vi "1B_HiStim_AnalyzePulseTrain.vi"(0 "Waveform In":waveform(dbl)={"t0"=timestamp(3433165898.5470004 s since 1904-01-01), "dt"=1e-05, "Y"=array[4250 elements]}, 5 "Repetitions in the Input Waveform":i32, 7 "Pulse Characteristics":T1={"Pulses per Cycle"=2, "Load Resistance (Ohms)"=750.0, "Krec Value"=2, "Recovery Mode (T=Active)"=TRUE, "Target Stim Currents (Amps)"=[]} {"Target Stim Currents (Amps)" format="%#_6p"}) -> (2 "Avg. CBC Width":dbl format="%0.6f", 3 "Avg. CBC Amplitude":dbl format="%0.2f", 4 "Stim PW":dbl[](array[numeric]), 6 "Stim Amplitude":dbl[](array[numeric]), 8 "Interphase Delay":dbl[](array[numeric]), 10 "Recovery PW":dbl[](array[numeric]), 12 "Waveform Parameters":T2 {"Frequency" format="%#_6p"; "Avg CBC Width" format="%#_6p"; "Avg. CBC Holdoff" format="%#_6p"; "Stim Pulse Width" format="%^#_6g"; "Interphase Delay" format="%#_6p"; "Recovery PW" format="%#_6p"; "Recovery Holdoff" format="%#_6p"; "Stim Amplitude" format="%^#_6g"; "Recovery Amplitude" format="%#_6p"}, 13 "Frequency":dbl, 14 "Recovery Holdoff":dbl[](array[numeric]), 15 "Recovery Amplitude":dbl[](array[numeric]))   [LabVIEW 2010]
uses:
  <vilib>/measure/mamon.llb/Trigger Detection for 1 Channel.vi
  <vilib>/measure/NI_MAPro.lvlib
  <vilib>/Analysis/NI_AALBase.lvlib
panel:
  in  "View":enum32{"View All", "Graph Only"}(tab)
  out "Waveform in ( graph )":waveform(dbl)(graph)
  out "Normalized Waveform":waveform(dbl)(graph)
  out "Offset":dbl
  out "Eq. Freq ( Hz )":dbl format="%#_6p"
  out "Current in amps":waveform(dbl)(graph)
  out "Time2 - Time1 ( sec )":dbl format="%#_6p"
  out "index":i32
  # "Remove idle voltage offset\n( if applicable )"
  # "The input waveform should be a capture of the STIM chip output\n(before the cap) when the output is held at 1/2 HVDD by the\nLoad Resistance.  This ensures that passive recovery and CBC\npulses are captured, because they look like pulses pulled to GND."
  # "The elements in these arrays correspond to the pulses per cycle.\nThey are the averages over all the repetitions in the waveform."
  # "Enter Target Current\nfor each in array below"
  # "1. Update Cursor Positions\n2. Turn off X Autoscaling\n3. Run this VI again"
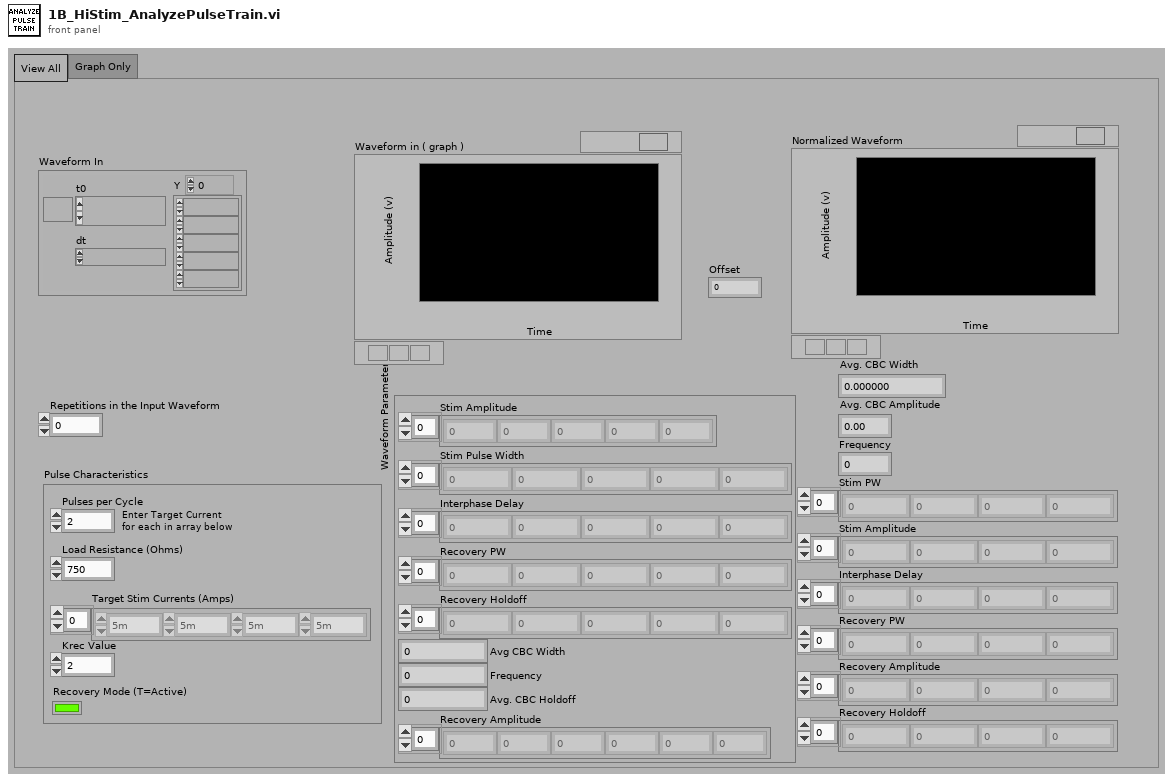
[diagram p1: front panel]
types:
  T1 = cluster{"Pulses per Cycle":i32, "Load Resistance (Ohms)":dbl, "Krec Value":i32, "Recovery Mode (T=Active)":bool, "Target Stim Currents (Amps)":dbl[]}
  T2 = cluster{"Stim Amplitude":dbl[], "Stim Pulse Width":dbl[], "Interphase Delay":dbl[], "Recovery PW":dbl[], "Recovery Holdoff":dbl[], "Avg CBC Width":dbl, "Frequency":dbl, "Avg. CBC Holdoff":dbl, "Recovery Amplitude":dbl[]}
  T3 = cluster{"trigger slope":u16, "Trigger Level":dbl}[]
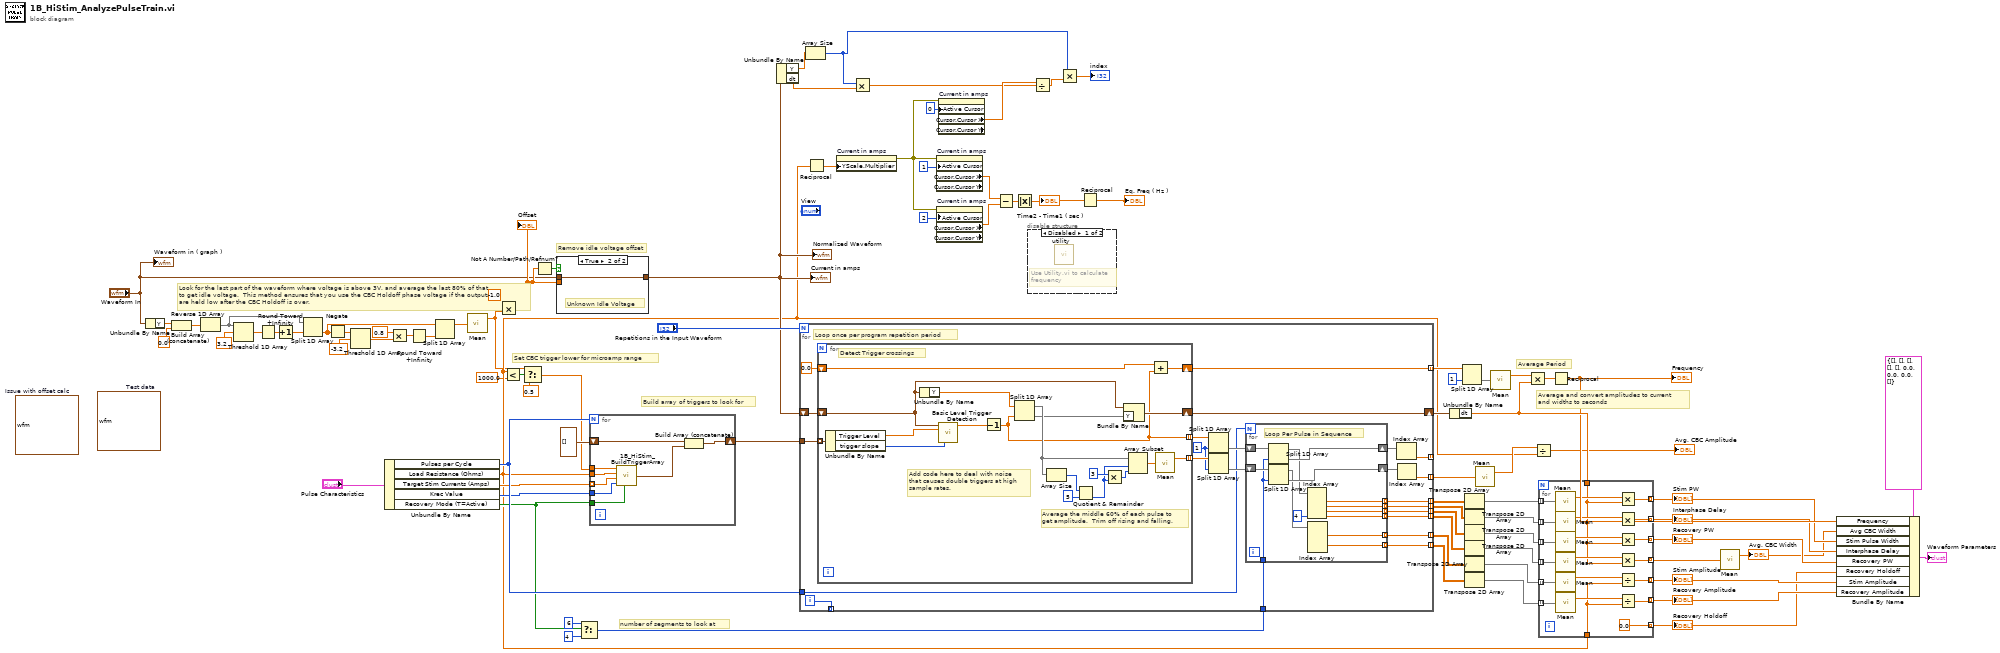
[diagram p0: block diagram]
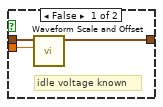
[diagram p3: hidden frame]
diagram:
  (unwired) waveform(dbl) {"t0"=timestamp(3458836317.3280005 s since 1904-01-01), "dt"=1.428e-05, "Y"=array[4000 elements]}  # Issue with offset calc
  (unwired) waveform(dbl) {"t0"=timestamp(3418839276.250478 s since 1904-01-01), "dt"=1e-06, "Y"=[5.0, 5.0, 9.0, 9.0, 9.0, 9.0, 9.0, 9.0, 9.0, 9.0, 5.0, 5.0, 5.0, 3.0, 3.0, 3.0, 3.0, 3.0, 3.0, 3.0, 3.0, 3.0, 3.0, 3.0, 3.0, 3.0, 3.0, 3.0, 3.0, 5.0, 5.0, 5.0, 5.0, 8.0, 8.0, 8.0, 8.0, 8.0, 8.0, 8.0, 8.0, 5.0, 5.0, 5.0, 3.0, 3.0, 3.0, 3.0, 3.0, 3.0, 3.0, 3.0, 3.0, 3.0, 3.0, 3.0, 3.0, 3.0, 3.0, 3.0, 5.0, 5.0, 5.0, 5.0, 0.0, 0.0, 0.0, 0.0, 0.0, 5.0, 5.0, 5.0, 5.0, 5.0, 5.0, 5.0, 5.0, 5.0, 5.0, 5.0, 5.0, 5.0, 5.0, 5.0, 5.0, 5.0, 5.0, 5.0, 5.0, 5.0, 5.0, 5.0, 5.0, 5.0, 5.0, 5.0, 5.0, 5.0, 5.0, 5.0, 5.0, 5.0, 9.0, 9.0, 9.0, 9.0, 9.0, 9.0, 9.0, 9.0, 5.0, 5.0, 5.0, 3.0, 3.0, 3.0, 3.0, 3.0, 3.0, 3.0, 3.0, 3.0, 3.0, 3.0, 3.0, 3.0, 3.0, 3.0, 3.0, 5.0, 5.0, 5.0, 5.0, 8.0, 8.0, 8.0, 8.0, 8.0, 8.0, 8.0, 8.0, 5.0, 5.0, 5.0, 3.0, 3.0, 3.0, 3.0, 3.0, 3.0, 3.0, 3.0, 3.0, 3.0, 3.0, 3.0, 3.0, 3.0, 3.0, 3.0, 5.0, 5.0, 5.0, 5.0, 0.0, 0.0, 0.0, 0.0, 0.0, 5.0, 5.0, 5.0, 5.0, 5.0, 5.0, 5.0, 5.0, 5.0, 5.0, 5.0, 5.0, 5.0, 5.0, 5.0, 5.0, 5.0, 5.0, 5.0, 5.0, 5.0, 5.0, 5.0, 5.0, 5.0, 5.0, 5.0, 5.0, 5.0, 5.0, 5.0, 5.0, 5.0, 9.0, 9.0, 9.0, 9.0, 9.0, 9.0, 9.0, 9.0, 5.0, 5.0, 5.0, 3.0, 3.0, 3.0, 3.0, 3.0, 3.0, 3.0, 3.0, 3.0, 3.0, 3.0, 3.0, 3.0, 3.0, 3.0, 3.0, 5.0, 5.0, 5.0, 5.0, 8.0, 8.0, 8.0, 8.0, 8.0, 8.0, 8.0, 8.0, 5.0, 5.0, 5.0, 3.0, 3.0, 3.0, 3.0, 3.0, 3.0, 3.0, 3.0, 3.0, 3.0, 3.0, 3.0, 3.0, 3.0, 3.0, 3.0, 5.0, 5.0, 5.0, 5.0, 0.0, 0.0, 0.0, 0.0, 0.0, 5.0, 5.0, 5.0, 5.0, 5.0, 5.0, 5.0, 5.0, 5.0, 5.0, 5.0, 5.0, 5.0, 5.0, 5.0, 5.0, 5.0, 5.0, 5.0, 5.0, 5.0, 5.0, 5.0, 5.0, 5.0, 5.0, 5.0, 5.0, 5.0, 5.0, 5.0, 5.0, 5.0, 9.0, 9.0, 9.0, 9.0, 9.0, 9.0, 9.0, 9.0, 5.0, 5.0, 5.0, 3.0, 3.0, 3.0, 3.0, 3.0, 3.0, 3.0, 3.0, 3.0, 3.0, 3.0, 3.0, 3.0, 3.0, 3.0, 3.0, 5.0, 5.0, 5.0, 5.0, 8.0, 8.0, 8.0, 8.0, 8.0, 8.0, 8.0, 8.0, 5.0, 5.0, 5.0, 3.0, 3.0, 3.0, 3.0, 3.0, 3.0, 3.0, 3.0, 3.0, 3.0, 3.0, 3.0, 3.0, 3.0, 3.0, 3.0, 5.0, 5.0, 5.0, 5.0, 0.0, 0.0, 0.0, 0.0, 0.0, 5.0, 5.0, 5.0, 5.0, 5.0, 5.0, 5.0, 5.0, 5.0, 5.0, 5.0, 5.0, 5.0, 5.0, 5.0, 5.0, 5.0, 5.0, 5.0, 5.0, 5.0, 5.0, 5.0, 5.0, 5.0, 5.0, 5.0, 5.0, 5.0, 5.0, 5.0, 5.0, 5.0, 9.0, 9.0, 9.0, 9.0, 9.0, 9.0, 9.0, 9.0, 5.0, 5.0, 5.0, 3.0, 3.0, 3.0, 3.0, 3.0, 3.0, 3.0, 3.0, 3.0, 3.0, 3.0, 3.0, 3.0, 3.0, 3.0, 3.0, 5.0, 5.0, 5.0, 5.0, 8.0, 8.0, 8.0, 8.0, 8.0, 8.0, 8.0, 8.0, 5.0, 5.0, 5.0, 3.0, 3.0, 3.0, 3.0, 3.0, 3.0, 3.0, 3.0, 3.0, 3.0, 3.0, 3.0, 3.0, 3.0, 3.0, 3.0, 5.0, 5.0, 5.0, 5.0, 0.0, 0.0, 0.0, 0.0, 0.0, 5.0, 5.0, 5.0, 5.0, 5.0, 5.0, 5.0, 5.0, 5.0, 5.0, 5.0, 5.0, 5.0, 5.0, 5.0, 5.0, 5.0, 5.0, 5.0, 5.0, 5.0, 5.0, 5.0, 5.0, 5.0, 5.0, 5.0, 5.0, 5.0, 5.0, 5.0, 5.0, 5.0, 5.0]}  # Test data
  # "Set CBC trigger lower for microamp range"
  # "number of segments to look at"
  # "Look for the last part of the waveform where voltage is above 3V, and average the last 80% of that\nto get idle voltage.  This method ensures that you use the CBC Holdoff phase voltage if the outputs\nare held low after the CBC Holdoff is over."
  # "Average Period"
  # "Average and convert amplitudes to current\nand widths to seconds"
  # "Build array of triggers to look for"
  # "Remove idle voltage offset"
  n1 = Unbundle By Name("Waveform In") -> ("Y"=w9:dbl[])
  n2 = Build Array (concatenate)(w9, 0.0 ("y")) -> (w8:dbl[])
  n3 = Reverse 1D Array(array=w8) -> (reversed array=w7:dbl[])
  n4 = Threshold 1D Array(2:3.2 ("y"), 3:w7) -> (0:w52:dbl)  [unwired: 1 in]
  n5 = Round Toward +Infinity(x=w52) -> (ceil(x): smallest int >= x=w51:dbl)
  n6 = Increment(x=w51) -> (x+1=w44:dbl)
  n7 = Split 1D Array(array=w7, index=w44) -> (second subarray=w32:dbl[])  [unwired: 1 out]
  n8 = Negate(x=w32) -> (-x=w49:dbl[])
  n9 = Threshold 1D Array(2:-3.2 ("y"), 3:w49) -> (0:w48:dbl)  [unwired: 1 in]
  n10 = Unbundle By Name("Pulse Characteristics") -> ("Pulses per Cycle"=w73:i32, "Load Resistance (Ohms)"=w6:dbl, "Target Stim Currents (Amps)"=w18:dbl[], "Krec Value"=w72:i32, "Recovery Mode (T=Active)"=w39:bool)
  n11 = Multiply(x=0.8, y=w48) -> (x*y=w46:dbl)
  n12 = Round Toward +Infinity(x=w46) -> (ceil(x): smallest int >= x=w45:dbl)
  n13 = Split 1D Array(array=w32, index=w45) -> (first subarray=w31:dbl[])  [unwired: 1 out]
  n14 = call <vilib>:"Mean.vi"("X"=w31) -> ("mean"=w3:dbl)  [unwired: 1 out]
  n15 = Multiply(x=-1.0, y=w3) -> (x*y=w34:dbl)
  "Offset" <- w34
  n16 = Less?(x=w6, y=1000.0) -> (x < y?=w4:bool)
  n17 = Select(t=w3, s=w4, f=0.5) -> (s? t:f=w2:dbl)
  n18 = Not A Number/Path/Refnum?(number/path/refnum=w34) -> (NaN/Path/Refnum?=w33:bool)
  n19 = case shown="True" w33 {
    tunnel: [w91 w92] -> w17
    tunnel: "Waveform In" -> [w90 w92]
    tunnel: w34 -> [w89 _]
    frame False {
      # "idle voltage known"
      n20 = call <vilib>:"Waveform Scale and Offset.vi"("offset"=w89, "waveform in"=w90) -> ("waveform out"=w91:waveform(dbl))  [unwired: 8 in, 1 out]
    }
    frame True {
      # "Unknown Idle Voltage"
    }
  }
  "Normalized Waveform" <- w17
  "Current in amps" <- w17
  n21 = Select(t=6, s=w39, f=4 ("index")) -> (s? t:f=w37:i32)
  n22 = for {
    N: w73 -> [_]
    shift-right: [w100] -> w43
    shift-left: T3 [] -> [w99]
    tunnel: w2 -> [w98]
    tunnel: w39 -> [w97]
    tunnel: w6 -> [w96]
    tunnel: w18 -> [w95] mode=indexing
    tunnel: w72 -> [w94]
    n23 = call "1B_HiStim_BuildTriggerArray.vi"("CBC Trigger Level"=w98, "Load Resistance (Ohms)"=w96, "Target Stim Current (Amps)"=w95, "Krec Value"=w94, "Recovery Mode (T=Active)"=w97) -> ("Pulse Triggers"=w93:T3)
    n24 = Build Array (concatenate)(w99, w93) -> (w100:T3)
  }
  n25 = Unbundle By Name(w17) -> ("Y"=w13:dbl[], "dt"=w12:dbl)
  n26 = for {
    N: "Repetitions in the Input Waveform" -> [_]
    tunnel: w43 -> [w123]
    shift-right: [w119] -> w70
    shift-left: w17 -> [w122]
    tunnel: w73 -> [w116]
    tunnel: [w113] -> _ mode=indexing
    tunnel: [w112] -> w86 mode=indexing
    tunnel: [w111] -> w85 mode=indexing
    tunnel: [w110] -> w84 mode=indexing
    tunnel: [w109] -> w83 mode=indexing
    tunnel: [w108] -> w82 mode=indexing
    tunnel: [w107] -> w81 mode=indexing
    tunnel: [w106] -> w80 mode=indexing
    tunnel: [w103] -> w68 mode=indexing
    tunnel: w37 -> [w102]
    tunnel: [w101] -> _ mode=indexing
    i -> [w101]
    w120 = 1 ("index")
    # "Loop once per program repetition period"
    n27 = for {
      tunnel: w123 -> [w156] mode=indexing
      shift-right: [w143] -> w119
      shift-left: w122 -> [w139]
      tunnel: [w148] -> w121 mode=indexing
      tunnel: [w141] -> w104 mode=indexing
      shift-right: [w147] -> w103
      shift-left: 0.0 -> [w146]
      # "Add code here to deal with noise \nthat causes double triggers at high\nsample rates."
      # "Detect Trigger crossings"
      # "Average the middle 60% of each pulse to\nget amplitude.  Trim off rising and falling."
      n28 = Unbundle By Name(w156) -> ("Trigger Level"=w145:dbl, "trigger slope"=w144:u16)
      n29 = Unbundle By Name(w139) -> ("Y"=w140:dbl[])
      n30 = call-poly <vilib>:"Basic Level Trigger Detection.vi"("signal in"=w139, "level"=w145, "trigger slope"=w144) -> ("trigger location"=w138:dbl)  [unwired: 10 in, 2 out]
      n31 = Decrement(x=w138) -> (x-1=w141:dbl)
      n32 = Split 1D Array(array=w140, index=w141) -> (first subarray=w150:dbl[], second subarray=w142:dbl[])
      n33 = Array Size(array=w150) -> (size(s)=w155:i32)
      n34 = Quotient & Remainder(x=w155, y=5) -> (floor(x/y)=w152:i32)  [unwired: 1 out]
      n35 = Multiply(x=3, y=w152) -> (x*y=w151:i32)
      n36 = Bundle By Name(cluster=w139, "Y"=w142) -> (w143:waveform(dbl))
      n37 = Array Subset(array=w150, index=w152, length=w151) -> (w149:dbl[])
      n38 = Add(x=w146, y=w141) -> (x+y=w147:dbl)
      n39 = call <vilib>:"Mean.vi"("X"=w149) -> ("mean"=w148:dbl)  [unwired: 1 out]
    }
    n40 = Split 1D Array(array=w104, index=w120) -> (second subarray=w118:dbl[])  [unwired: 1 out]
    n41 = Split 1D Array(array=w121, index=w120) -> (second subarray=w117:dbl[])  [unwired: 1 out]
    n42 = for {
      N: w116 -> [_]
      shift-right: [w135] -> w115
      shift-left: w118 -> [w137]
      shift-right: [w134] -> w114
      shift-left: w117 -> [w136]
      tunnel: [w131] -> w111 mode=indexing
      tunnel: [w130] -> w110 mode=indexing
      tunnel: [w129] -> w109 mode=indexing
      tunnel: [w128] -> w108 mode=indexing
      tunnel: [w127] -> w107 mode=indexing
      tunnel: [w126] -> w106 mode=indexing
      tunnel: w102 -> [w125]
      # "Loop Per Pulse in Sequence"
      n43 = Split 1D Array(array=w137, index=w125) -> (first subarray=w133:dbl[], second subarray=w135:dbl[])
      n44 = Split 1D Array(array=w136, index=w125) -> (first subarray=w132:dbl[], second subarray=w134:dbl[])
      n45 = Index Array(array=w133, index #4=4 ("index")) -> (element #1=w131:dbl, element #2=w130:dbl, element #3=w129:dbl, element #4=w128:dbl)  [unwired: 3 in]
      n46 = Index Array(array=w132) -> (element #1=w127:dbl, element #3=w126:dbl)  [unwired: 4 in, 2 out]
    }
    n47 = Index Array(array=w115) -> (element=w113:dbl)  [unwired: 1 in]
    n48 = Index Array(array=w114) -> (element=w112:dbl)  [unwired: 1 in]
  }
  n49 = Array Size(array=w13) -> (size(s)=w11:i32)
  n50 = Reciprocal(x=w6) -> (1/x=w35:dbl)
  n51 = property on="Current in amps" class="WFGraph (strict)"("YScale.Multiplier"=w35) -> (error out=w20:errorcluster)  [unwired: 2 in, 1 out]
  n52 = Multiply(x=w11, y=w12) -> (x*y=w10:dbl)
  n53 = property on="Current in amps" class="WFGraph (strict)" props=["Active Cursor", "Cursor", "Cursor X", "Cursor", "Cursor Y"](error in=w20, "Active Cursor"=u32 1) -> ("Cursor.Cursor X"=w24:dbl)  [unwired: 1 in, 3 out]
  n54 = property on="Current in amps" class="WFGraph (strict)" props=["Active Cursor", "Cursor", "Cursor X", "Cursor", "Cursor Y"](error in=w20, "Active Cursor"=u32 2) -> ("Cursor.Cursor X"=w23:dbl)  [unwired: 1 in, 3 out]
  n55 = property on="Current in amps" class="WFGraph (strict)" props=["Active Cursor", "Cursor", "Cursor X", "Cursor", "Cursor Y"](error in=w20, "Active Cursor"=u32 0) -> ("Cursor.Cursor X"=w16:dbl)  [unwired: 1 in, 3 out]
  n56 = Subtract(x=w24, y=w23) -> (x-y=w25:dbl)
  n57 = Absolute Value(x=w25) -> (abs(x)=w22:dbl)
  "Time2 - Time1 ( sec )" <- w22
  n58 = disable-structure shown="Disabled" {
    frame Disabled {
      # "Use Utility.vi to calculate\nfrequency"
      n59 = call "utility.vi"() -> ()  [unwired: 12 in]
    }
    frame Enabled {
    }
  }
  n60 = Divide(x=w16, y=w10) -> (x/y=w15:dbl)
  n61 = Multiply(x=w11, y=w15) -> (x*y=→"index":dbl)
  n62 = Reciprocal(x=w22) -> (1/x=→"Eq. Freq ( Hz )":dbl)
  n63 = Unbundle By Name(w70) -> ("dt"=w65:dbl)
  n64 = Split 1D Array(array=w68, index=1) -> (second subarray=w67:dbl[])  [unwired: 1 out]
  n65 = Transpose 2D Array(2D array=w85) -> (transposed array=w79:dbl[][])
  n66 = Transpose 2D Array(2D array=w84) -> (transposed array=w78:dbl[][])
  n67 = Transpose 2D Array(2D array=w83) -> (transposed array=w77:dbl[][])
  n68 = Transpose 2D Array(2D array=w82) -> (transposed array=w76:dbl[][])
  n69 = Transpose 2D Array(2D array=w81) -> (transposed array=w75:dbl[][])
  n70 = Transpose 2D Array(2D array=w80) -> (transposed array=w74:dbl[][])
  n71 = call <vilib>:"Mean.vi"("X"=w86) -> ("mean"=w69:dbl)  [unwired: 1 out]
  n72 = call <vilib>:"Mean.vi"("X"=w67) -> ("mean"=w66:dbl)  [unwired: 1 out]
  n73 = Multiply(x=w66, y=w65) -> (x*y=w64:dbl)
  n74 = Divide(x=w69, y=w6) -> (x/y=→"Avg. CBC Amplitude":dbl)
  n75 = for {
    tunnel: w79 -> [w177] mode=indexing
    tunnel: w78 -> [w176] mode=indexing
    tunnel: w77 -> [w175] mode=indexing
    tunnel: w76 -> [w174] mode=indexing
    tunnel: w75 -> [w173] mode=indexing
    tunnel: w74 -> [w172] mode=indexing
    tunnel: [w171] -> w59 mode=indexing
    tunnel: [w170] -> w58 mode=indexing
    tunnel: [w169] -> w57 mode=indexing
    tunnel: [w168] -> w41 mode=indexing
    tunnel: [w167] -> w56 mode=indexing
    tunnel: [w166] -> w55 mode=indexing
    tunnel: w65 -> [w159]
    tunnel: w6 -> [w158]
    tunnel: [0.0 ("Load Resistance (Ohms)")] -> w42 mode=indexing
    n76 = call <vilib>:"Mean.vi"("X"=w177) -> ("mean"=w164:dbl)  [unwired: 1 out]
    n77 = call <vilib>:"Mean.vi"("X"=w176) -> ("mean"=w163:dbl)  [unwired: 1 out]
    n78 = call <vilib>:"Mean.vi"("X"=w175) -> ("mean"=w162:dbl)  [unwired: 1 out]
    n79 = call <vilib>:"Mean.vi"("X"=w174) -> ("mean"=w161:dbl)  [unwired: 1 out]
    n80 = call <vilib>:"Mean.vi"("X"=w173) -> ("mean"=w160:dbl)  [unwired: 1 out]
    n81 = call <vilib>:"Mean.vi"("X"=w172) -> ("mean"=w165:dbl)  [unwired: 1 out]
    n82 = Multiply(x=w164, y=w159) -> (x*y=w171:dbl)
    n83 = Multiply(x=w163, y=w159) -> (x*y=w170:dbl)
    n84 = Multiply(x=w162, y=w159) -> (x*y=w169:dbl)
    n85 = Multiply(x=w161, y=w159) -> (x*y=w168:dbl)
    n86 = Divide(x=w160, y=w158) -> (x/y=w167:dbl)
    n87 = Divide(x=w165, y=w158) -> (x/y=w166:dbl)
  }
  "Stim PW" <- w59
  "Interphase Delay" <- w58
  "Recovery PW" <- w57
  "Recovery Holdoff" <- w42
  "Stim Amplitude" <- w56
  "Recovery Amplitude" <- w55
  n88 = Reciprocal(x=w64) -> (1/x=w61:dbl)
  "Frequency" <- w61
  n89 = call <vilib>:"Mean.vi"("X"=w41) -> ("mean"=w40:dbl)  [unwired: 1 out]
  "Avg. CBC Width" <- w40
  n90 = Bundle By Name(cluster=T2 {"Stim Amplitude"=[], "Stim Pulse Width"=[], "Interphase Delay"=[], "Recovery PW"=[], "Recovery Holdoff"=[], "Avg CBC Width"=0.0, "Frequency"=0.0, "Avg. CBC Holdoff"=0.0, "Recovery Amplitude"=[]} ("Pulse Train Parameters"), "Frequency"=w61, "Avg CBC Width"=w40, "Stim Pulse Width"=w59, "Interphase Delay"=w58, "Recovery PW"=w57, "Recovery Holdoff"=w42, "Stim Amplitude"=w56, "Recovery Amplitude"=w55) -> (→"Waveform Parameters":T2)
  "Waveform in ( graph )" <- "Waveform In"
